vi "getSweepData.vi"(8 "error in (no error)":errorcluster, 11 "Instrument.LockinAPI in":refnum<class "Instrument.LockinAPI.lvclass">) -> (0 "error out":errorcluster, 2 "SweepData":T1, 3 "Instrument.LockinAPI out":refnum<class "Instrument.LockinAPI.lvclass">)   [LabVIEW 2019, in "Instrument.LockinAPI.lvclass"]
doc: "API to get the results of lockin calculation.\n\nIf address=\"\", this API reads from localhost\nIf address is remote lockin, you need to add this computer to allowed whitelist on the lockin computer you are trying to access."
uses:
  Instrument.LockinAPI.lvclass
  C:/Users/patrick/Documents/GitHub/Instrument-Framework/lvsrc/Instrument/Instrument.lvclass
  Typedefs/LockinAPI.SweepData--Cluster.ctl
  Typedefs/LockinAPI.Commands--Enum.ctl
  c571ce1c-8d9e-4ac0-93b7-96f20f760cb3.vi
  c571ce1c-8d9e-4ac0-93b7-96f20f760cb3.vi/c08b6385-ef0e-4fe9-8886-a06e87bde4d0.vi
  c571ce1c-8d9e-4ac0-93b7-96f20f760cb3.vi/c08b6385-ef0e-4fe9-8886-a06e87bde4d0.vi/8f6ed12d-b05c-4d7d-8334-9f2c757b5755.vi
  c571ce1c-8d9e-4ac0-93b7-96f20f760cb3.vi/c08b6385-ef0e-4fe9-8886-a06e87bde4d0.vi/42c2e330-ee3c-4561-aa72-2c07bdf8c65a.vi
  Instrument/Protected/Validate API method.vi
  Instrument/Private/Get RC Connection Status.vi
  Instrument/API/Send and Receive.vi
  <vilib>/Utility/Data Type/Get Type Information.vi
  <vilib>/JDP Science/JSONtext/JSON text to Variant.vi
  <vilib>/JDP Science/JSONtext/LVClass Serializer/JSONtext LVClass Serializer.lvclass
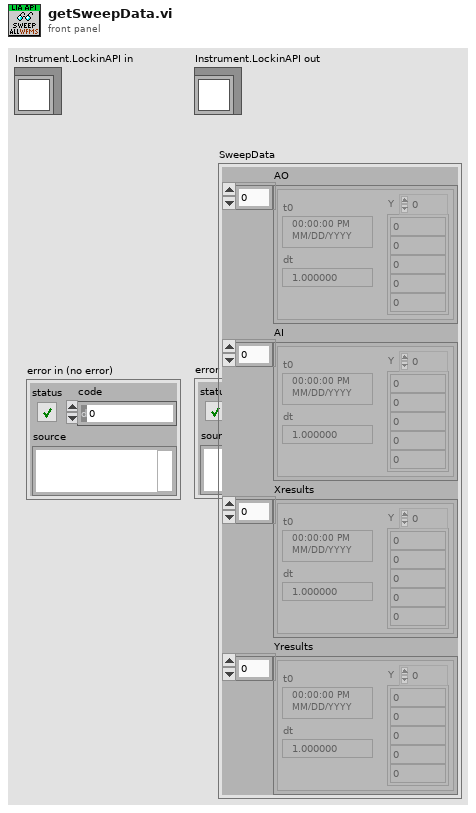
[diagram p1: front panel]
types:
  T1 = typedef "Instrument.LockinAPI.lvclass/LockinAPI.SweepData--Cluster.ctl" = cluster{"AO":waveform(dbl)[], "AI":waveform(dbl)[], "Xresults":waveform(dbl)[], "Yresults":waveform(dbl)[]}
  T2 = typedef "Instrument.LockinAPI.lvclass/LockinAPI.Commands--Enum.ctl" = enum16{"setAI", "setAO", "setAO_Amplitude", "setAO_DC", "setAO_Frequency", "setAO_Phase", "setAO_Function", "setAO_I+", "setREF", "setREF_Frequency", "setREF_Phase", "setREF_TC", "setREF_Roll-Off", "setDAQ", "setSampling", "setOffset", "setState", "getState", "getAO", "getAI", "getResults", "getSampling", "getAOconfig", "getREFconfig", "setInputGain", "setOutputGain", "getInputGain", "getOutputGain", "setSamplingMode", "getSamplingMode", "setSweep", "setSweepTime", "setSweepTable", "getStatus", "getSweepResults", "getSweepWaveforms", "startSweep", "stopSweep", "setAUX", "getAUX"}
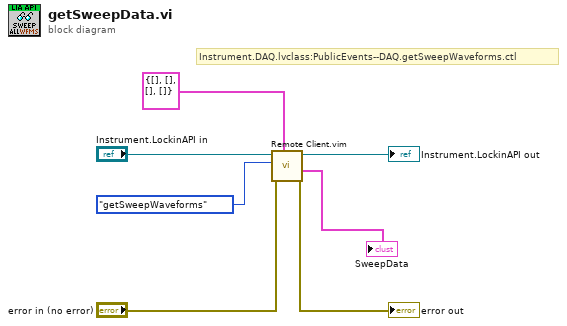
[diagram p0: block diagram]
diagram:
  # "Instrument.DAQ.lvclass:PublicEvents--DAQ.getSweepWaveforms.ctl"
  n1 = call "Remote Client.vim"("Data Out type"=T1 {"AO"=[], "AI"=[], "Xresults"=[], "Yresults"=[]} ("sweepData"), "error in (no error)"="error in (no error)", "Command in"=LockinAPI.Commands--Enum."getSweepWaveforms" ("Command"), "Instrument in"="Instrument.LockinAPI in") -> ("error out"=→"error out":errorcluster, "Data out"=→"SweepData":T1, "Instrument out"=→"Instrument.LockinAPI out":refnum<class "Instrument.LockinAPI.lvclass">)  [unwired: 4 in, 1 out]
